vi "Regular Waves.vi"(0 "Run":bool, 1 "Wave Period":dbl(slide)=1.0 min=0.5 max=5.0 step=0.01 scale=0.5..5.0 scale format="%.1f", 2 "Wave Height":dbl(slide)=0.1 min=0.0 step=0.001 scale=0.0..0.15606733627984637 scale format="%.3f") -> ()   [LabVIEW 2012]
uses:
  <vilib>/DAQmx/write.llb/DAQmx Write (Analog 1D DBL 1Chan NSamp).vi
  <vilib>/DAQmx/write.llb/DAQmx Write (Analog 1D DBL NChan 1Samp).vi
  <vilib>/DAQmx/write.llb/DAQmx Write (Analog 2D DBL NChan NSamp).vi
  <vilib>/DAQmx/read.llb/DAQmx Read (Analog 2D DBL NChan NSamp).vi
  <vilib>/DAQmx/write.llb/DAQmx Write (Analog DBL 1Chan 1Samp).vi
  <vilib>/DAQmx/create/channels.llb/DAQmx Create Channel (AO-Voltage-Basic).vi
  <vilib>/DAQmx/configure/timing.llb/DAQmx Timing (Use Waveform).vi
  <vilib>/DAQmx/create/channels.llb/DAQmx Create Channel (AI-Voltage-Basic).vi
  <vilib>/DAQmx/configure/timing.llb/DAQmx Timing (Sample Clock).vi
  <vilib>/Analysis/1siggen.llb/Ramp Pattern by Samples.vi
  <vilib>/DAQmx/miscellaneous.llb/DAQmx Fill In Error Info.vi
  <vilib>/Analysis/NI_AALBase.lvlib
panel:
  out "Waveform Chart":dbl[][](graph)
  in  "Measure Waves":bool
  in  "Settings":bool
  in  "Power":bool
  out "Buffer Size":i32=4000
  # "Regular Wave Generator"
  # "s"
  # "m"
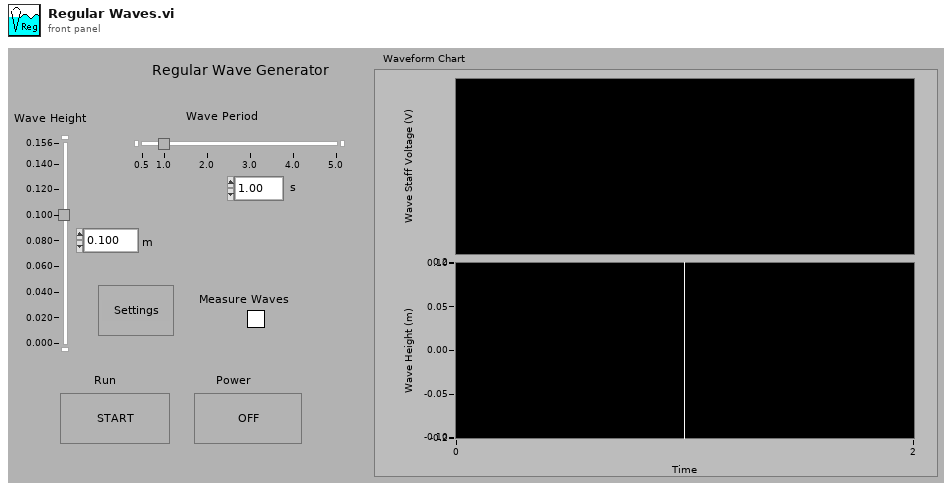
[diagram p1: front panel]
types:
  T1 = cluster{"Output Device":i16, "Output Channel":string, "Sampling Rate (Hz)":dbl, "Input Device":i16, "Input Channel":string, "Input Offset (V)":dbl, "Input Calibration (m/V)":dbl, "Stroke Calibration (V/m)":dbl, "Paddle Height (m)":dbl, "Water Depth (m)":dbl, "Min Period":dbl, "Max Period":dbl, "Max 1/2 Piston Stroke":dbl, "Max H/L":dbl, "Max H/d":dbl}
  T2 = cluster{"Period":dbl, "Wave Height":dbl, "Phase Angle (rad)":dbl}
  T3 = cluster{"Sampling Rate":i32, "Water Depth":dbl, "Paddle Height":dbl}
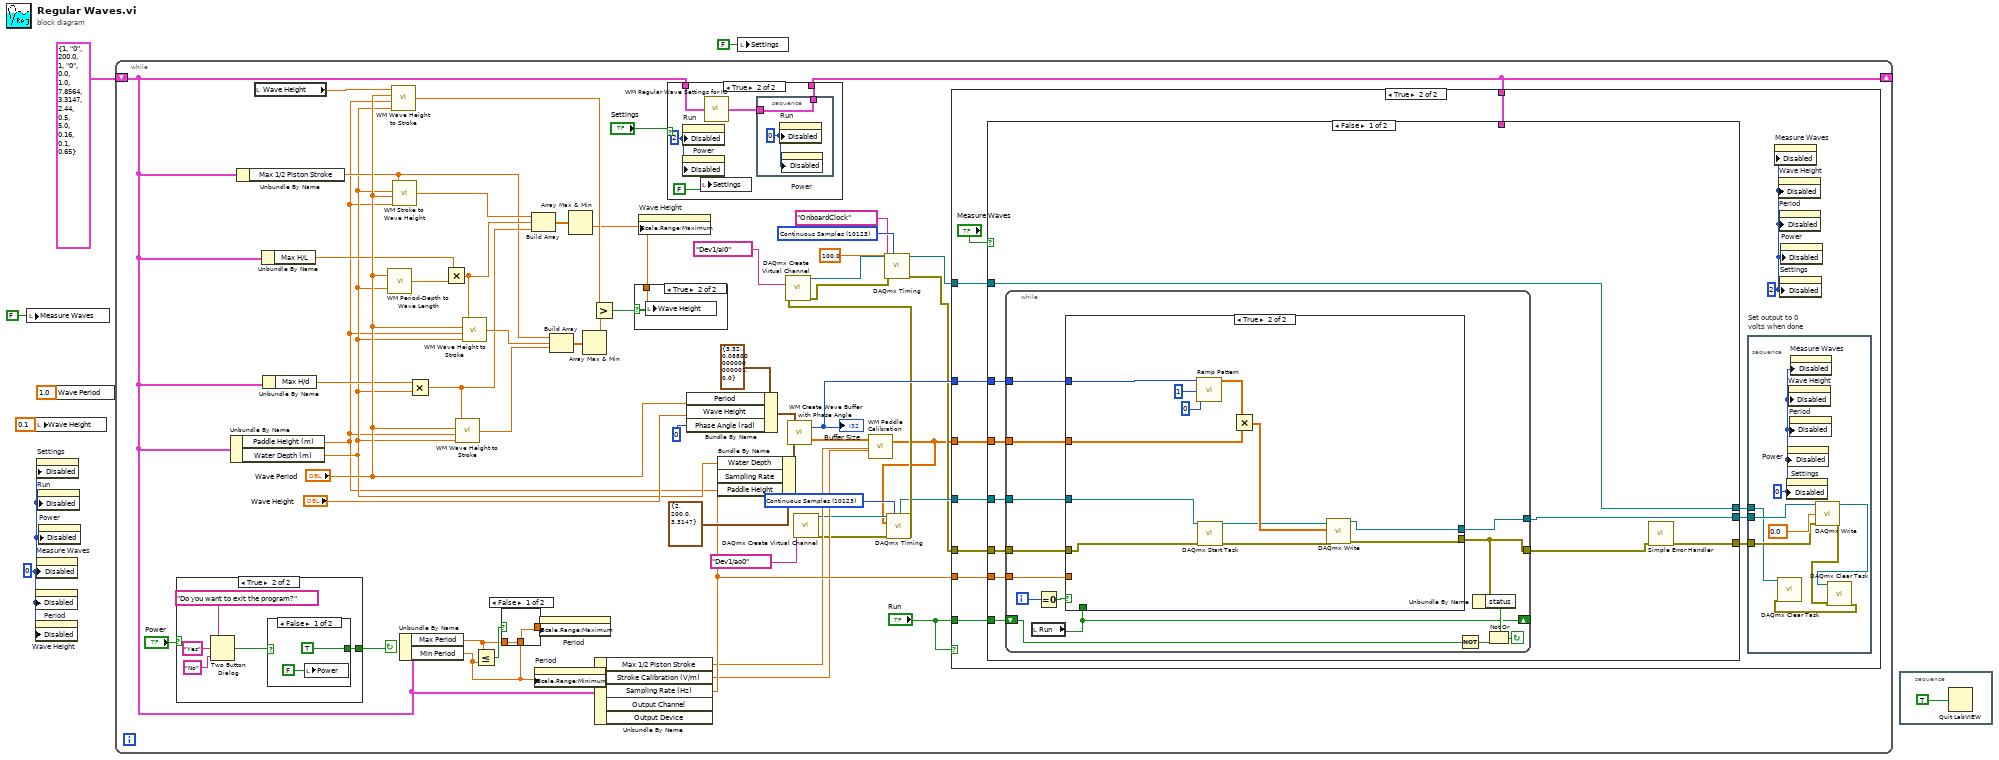
[diagram p0: block diagram]
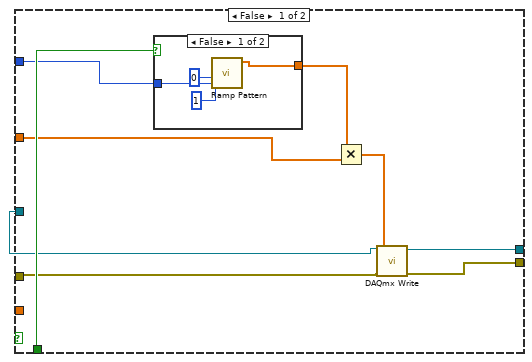
[diagram p3: hidden frame]
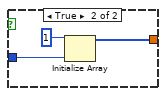
[diagram p4: hidden frame]
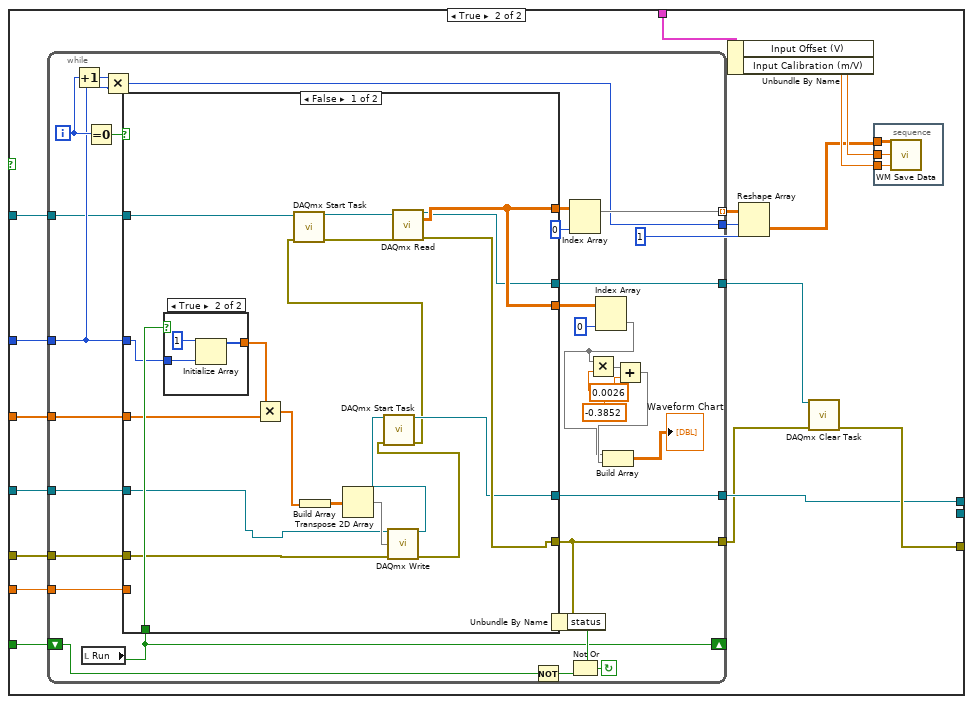
[diagram p5: hidden frame]
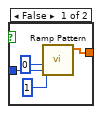
[diagram p6: hidden frame]
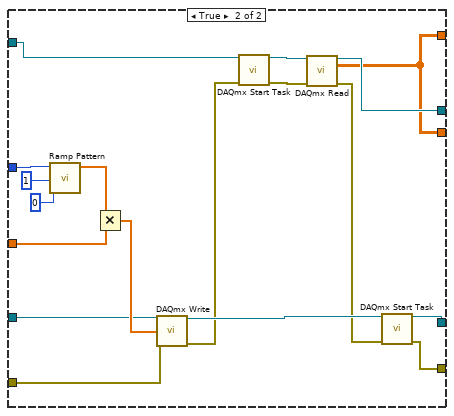
[diagram p7: hidden frame]
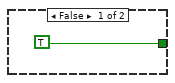
[diagram p9: hidden frame]
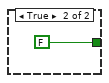
[diagram p10: hidden frame]
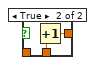
[diagram p11: hidden frame]
diagram:
  w2 = u8 0 ("Write Attribute")
  n1 = local write "Measure Waves"(FALSE ("Measure Waves")) -> ()
  n2 = local write "Wave Height"(0.1 ("Wave Height")) -> ()
  n3 = property on="Period" class="Slide (strict)"("Disabled"=w2) -> ()  [unwired: 2 in, 2 out]
  n4 = property on="Wave Height" class="Slide (strict)"("Disabled"=w2) -> ()  [unwired: 2 in, 2 out]
  n5 = property on="Measure Waves" class="Bool (strict)"("Disabled"=w2) -> ()  [unwired: 2 in, 2 out]
  n6 = property on="Settings" class="Bool (strict)"("Disabled"=w2) -> ()  [unwired: 2 in, 2 out]
  n7 = property on="Run" class="Bool (strict)"("Disabled"=w2) -> ()  [unwired: 2 in, 2 out]
  n8 = property on="Power" class="Bool (strict)"("Disabled"=w2) -> ()  [unwired: 2 in, 2 out]
  n9 = local write "Wave Period"(1.0 ("Period")) -> ()
  n10 = while {
    shift-left: T1 {"Output Device"=1, "Output Channel"="0", "Sampling Rate (Hz)"=200.0, "Input Device"=1, "Input Channel"="0", "Input Offset (V)"=0.0, "Input Calibration (m/V)"=1.0, "Stroke Calibration (V/m)"=7.8564, "Paddle Height (m)"=3.3147, "Water Depth (m)"=2.44, "Min Period"=0.5, "Max Period"=5.0, "Max 1/2 Piston Stroke"=0.16, "Max H/L"=0.1, "Max H/d"=0.65} ("Settings") -> [w27]
    shift-right: [w22] -> _
    stop <- w47 continue-if-true
    w9 = 10123 items=["Finite Samples"=10178, "Continuous Samples"=10123, "Hardware Timed Single Point"=12522] ("sample mode")
    w15 = 10123 items=["Finite Samples"=10178, "Continuous Samples"=10123, "Hardware Timed Single Point"=12522] ("sample mode")
    n11 = case shown="True" "Power" {
      tunnel: [TRUE w238] -> w47
      frame False {
      }
      frame True {
        n12 = Two Button Dialog(message="Do you want to exit the program?", 1:"No" ("F button name (\"Cancel\")"), 2:"Yes" ("T button name (\"OK\")")) -> (T button?=w239:bool)
        n13 = case shown="False" w239 {
          tunnel: [TRUE FALSE] -> w238
          frame False {
            n14 = local write "Power"(FALSE ("Power")) -> ()
          }
          frame True {
          }
        }
      }
    }
    n15 = Unbundle By Name(w27) -> ("Paddle Height (m)"=w30:dbl, "Water Depth (m)"=w31:dbl)
    n16 = Unbundle By Name(w27) -> ("Max 1/2 Piston Stroke"=w34:dbl)
    n17 = local read "Wave Height"() -> (w50:dbl)
    n18 = Unbundle By Name(w27) -> ("Max H/L"=w33:dbl)
    n19 = Unbundle By Name(w27) -> ("Max H/d"=w32:dbl)
    n20 = call "WM Period-Depth to Wave Length.vi"("Water Depth"=w31, "Period"="Wave Period") -> ("WaveLength"=w39:dbl)
    n21 = call "WM Wave Height to Stroke.vi"("Water Depth (m)"=w31, "Flap Height (m)"=w30, "Wave Period (s)"="Wave Period", "Wave Height (m)"=w50) -> ("Flap Amplitude (from x=0) (m)"=w59:dbl)
    n22 = call "WM Stroke to Wave Height.vi"("Paddle Height (m)"=w30, "Wave Period (s)"="Wave Period", "Water Depth (m)"=w31, "Flap Amplitude from x=0 (m)"=w34) -> ("Wave Height (m)"=w54:dbl)
    n23 = Unbundle By Name(w27) -> ("Max Period"=w26:dbl, "Min Period"=w25:dbl)
    n24 = Multiply(x=w32, y=w31) -> (x*y=w38:dbl)
    n25 = Multiply(x=w33, y=w39) -> (x*y=w55:dbl)
    n26 = call "WM Wave Height to Stroke.vi"("Water Depth (m)"=w31, "Flap Height (m)"=w30, "Wave Period (s)"="Wave Period", "Wave Height (m)"=w38) -> ("Flap Amplitude (from x=0) (m)"=w53:dbl)
    n27 = call "WM Wave Height to Stroke.vi"("Water Depth (m)"=w31, "Flap Height (m)"=w30, "Wave Period (s)"="Wave Period", "Wave Height (m)"=w55) -> ("Flap Amplitude (from x=0) (m)"=w52:dbl)
    n28 = Less Or Equal?(x=w26, y=w25) -> (x <= y?=w60:bool)
    n29 = case shown="False" w60 {
      tunnel: w25 -> [_ w248]
      tunnel: [w246 w247] -> w49
      tunnel: w26 -> [w246 _]
      frame False {
      }
      frame True {
        n30 = Increment(x=w248) -> (x+1=w247:dbl)
      }
    }
    n31 = Build Array(w54, w55, w38) -> (w58:dbl[])
    n32 = property on="Period" class="Slide (strict)"("Scale.Range:Minimum"=w25) -> ()  [unwired: 2 in, 2 out]
    n33 = property on="Period" class="Slide (strict)"("Scale.Range:Maximum"=w49) -> ()  [unwired: 2 in, 2 out]
    n34 = Build Array(w34, w52, w53) -> (w57:dbl[])
    n35 = Array Max & Min(array=w58) -> (min value=w51:dbl)  [unwired: 3 out]
    n36 = Array Max & Min(array=w57) -> (min value=w56:dbl)  [unwired: 3 out]
    n37 = Greater?(x=w59, y=w56) -> (0:w61:bool)
    n38 = Unbundle By Name(w27) -> ("Max 1/2 Piston Stroke"=w29:dbl, "Stroke Calibration (V/m)"=w28:dbl, "Sampling Rate (Hz)"=w35:dbl)  [unwired: 2 out]
    n39 = case shown="True" w61 {
      tunnel: w51 -> [_ w249]
      frame False {
      }
      frame True {
        n40 = local write "Wave Height"(w249) -> ()
      }
    }
    n41 = property on="Wave Height" class="Slide (strict)"("Scale.Range:Maximum"=w51) -> ()  [unwired: 2 in, 2 out]
    n42 = case shown="True" "Settings" {
      tunnel: w27 -> [w229 w234]
      tunnel: [w229 w232] -> w22
      frame False {
      }
      frame True {
        w230 = u8 2 ("Write Attribute")
        n43 = property on="Run" class="Bool (strict)"("Disabled"=w230) -> ()  [unwired: 2 in, 2 out]
        n44 = property on="Power" class="Bool (strict)"("Disabled"=w230) -> ()  [unwired: 2 in, 2 out]
        n45 = local write "Settings"(FALSE ("Settings")) -> ()
        n46 = call "WM Regular Wave Settings for IO.vi"("Settings"=w234) -> ("Settings Output"=w233:T1)
        n47 = stacked-sequence {
          tunnel: w233 -> [w236]
          tunnel: [w236] -> w232
          frame #0 {
            w235 = u8 0 ("Write Attribute")
            n48 = property on="Run" class="Bool (strict)"("Disabled"=w235) -> ()  [unwired: 2 in, 2 out]
            n49 = property on="Power" class="Bool (strict)"("Disabled"=w235) -> ()  [unwired: 2 in, 2 out]
          }
        }
      }
    }
    n50 = Bundle By Name(cluster=T2 {"Period"=3.32, "Wave Height"=0.08800000000000001, "Phase Angle (rad)"=0.0} ("Sine Paramaters"), "Period"="Wave Period", "Wave Height"="Wave Height", "Phase Angle (rad)"=0) -> (w42:T2)
    n51 = Bundle By Name(cluster=T3 {"Sampling Rate"=2, "Water Depth"=200.0, "Paddle Height"=3.3147} ("Buffer Info"), "Water Depth"=w31, "Sampling Rate"=w35, "Paddle Height"=w30) -> (w44:T3)
    n52 = call "WM Create Wave Buffer with Phase Angle.vi"("Buffer Info"=w44, "Sine Paramaters"=w42) -> ("Output"=w46:dbl[], "Buffer Size"=w24:i32)
    "Buffer Size" <- w24
    n53 = call-poly <vilib>:"DAQmx Create Virtual Channel.vi"("physical channels"=tag "Dev1/ao0") -> ("task out"=w19:refnum<k21>, "error out"=w18:errorcluster)  [unwired: 13 in]
    n54 = call "WM Paddle Calibration.vi"("Stroke Calibration (V/m)"=w28, "Max 1/2 Piston Stroke (m)"=w29, "Input Stroke Distance (m)"=w46) -> ("Output Voltage"=w7:dbl[])  [unwired: 1 in, 1 out]
    n55 = call-poly <vilib>:"DAQmx Timing.vi"("task/channels in"=w19, "sample mode"=w15, "waveform"=w7, "error in"=w18) -> ("task out"=w16:refnum<k21>, "error out"=w17:errorcluster)  [unwired: 10 in]
    n56 = call-poly <vilib>:"DAQmx Create Virtual Channel.vi"("physical channels"=tag "Dev1/ai0", "error in"=w17) -> ("task out"=w14:refnum<k21>, "error out"=w11:errorcluster)  [unwired: 12 in]
    n57 = call-poly <vilib>:"DAQmx Timing.vi"("task/channels in"=w14, "sample mode"=w9, "rate"=100.0, "source"=tag "OnboardClock", "error in"=w11) -> ("task out"=w13:refnum<k21>, "error out"=w12:errorcluster)  [unwired: 9 in]
    n58 = case shown="True" "Run" {
      tunnel: w24 -> [_ w73]
      tunnel: "Run" -> [_ w72]
      tunnel: w7 -> [_ w71]
      tunnel: w35 -> [_ w70]
      tunnel: w22 -> [_ w67]
      tunnel: w16 -> [_ w66]
      tunnel: w12 -> [_ w65]
      tunnel: w13 -> [_ w64]
      frame False {
      }
      frame True {
        w68 = u8 2 ("Write Attribute")
        n59 = case shown="False" "Measure Waves" {
          tunnel: [w84 w129] -> w74
          tunnel: w73 -> [w83 w144]
          tunnel: w72 -> [w82 w142]
          tunnel: w71 -> [w81 w143]
          tunnel: w70 -> [w80 w141]
          tunnel: w67 -> [_ w140]
          tunnel: w66 -> [w79 w133]
          tunnel: w65 -> [w78 w132]
          tunnel: w64 -> [w77 w131]
          tunnel: [w77 w128] -> w63
          tunnel: [w75 _] -> w62
          frame False {
            n60 = while {
              tunnel: [w89] -> w76
              tunnel: w83 -> [w90]
              tunnel: w81 -> [w91]
              tunnel: w80 -> [w92]
              shift-left: w82 -> [w93]
              shift-right: [w88] -> _
              tunnel: w79 -> [w87]
              tunnel: w78 -> [w86]
              tunnel: [w85] -> w75
              i -> [w98]
              stop <- w94 continue-if-true
              n61 = local read "Run"() -> (w88:bool)
              n62 = Equal To 0?(x=w98) -> (x = 0?=w97:bool)
              n63 = case shown="True" w97 {
                tunnel: [w99 w115] -> w89
                tunnel: w92 -> [_ _]
                tunnel: w88 -> [w106 _]
                tunnel: w91 -> [w105 w122]
                tunnel: w90 -> [w104 w123]
                tunnel: w87 -> [w101 w120]
                tunnel: w86 -> [w100 w119]
                tunnel: [w103 w116] -> w85
                frame False {
                  n64 = case shown="False" w106 {
                    tunnel: [w111 w112] -> w107
                    tunnel: w104 -> [w108 w114]
                    frame False {
                      n65 = call-poly <vilib>:"Ramp Pattern.vi"("start"=1, "end"=0, "samples"=w108) -> ("Ramp Pattern"=w111:dbl[])  [unwired: 7 in, 1 out]
                    }
                    frame True {
                      n66 = Initialize Array(1, w114) -> (w112:i32[])
                    }
                  }
                  n67 = Multiply(x=w107, y=w105) -> (x*y=w102:dbl[])
                  n68 = call-poly <vilib>:"DAQmx Write.vi"("task/channels in"=w101, "data"=w102, "error in"=w100) -> ("task out"=w103:refnum<k21>, "error out"=w99:errorcluster)  [unwired: 10 in, 1 out]
                }
                frame True {
                  n69 = call-poly <vilib>:"Ramp Pattern.vi"("start"=0, "end"=1, "samples"=w123) -> ("Ramp Pattern"=w124:dbl[])  [unwired: 7 in, 1 out]
                  n70 = call <vilib>:"DAQmx Start Task.vi"("task/channels in"=w120, "error in"=w119) -> ("task out"=w118:refnum<k21>, "error out"=w117:errorcluster)  [unwired: 12 in]
                  n71 = Multiply(x=w124, y=w122) -> (x*y=w121:dbl[])
                  n72 = call-poly <vilib>:"DAQmx Write.vi"("task/channels in"=w118, "data"=w121, "error in"=w117) -> ("task out"=w116:refnum<k21>, "error out"=w115:errorcluster)  [unwired: 10 in, 1 out]
                }
              }
              n73 = Not(x=w93) -> (.not. x?=w95:bool)
              n74 = Unbundle By Name(w89) -> ("status"=w96:bool)
              n75 = Not Or(1:w95, 2:w96) -> (0:w94:bool)
            }
            n76 = call <vilib>:"Simple Error Handler.vi"("error in (no error)"=w76) -> ("error out"=w84:errorcluster)  [unwired: 4 in, 4 out]
          }
          frame True {
            n77 = while {
              tunnel: [w158] -> w135
              tunnel: [w163] -> w137 mode=indexing
              tunnel: [w165] -> w127
              tunnel: w144 -> [w159]
              tunnel: w143 -> [w167]
              tunnel: w141 -> [w168]
              shift-left: w142 -> [w169]
              shift-right: [w166] -> _
              tunnel: w133 -> [w149]
              tunnel: w132 -> [w148]
              tunnel: w131 -> [w147]
              tunnel: [w146] -> w128
              tunnel: [w145] -> w130
              i -> [w161]
              stop <- w170 continue-if-true
              n78 = Increment(x=w161) -> (x+1=w160:i32)
              n79 = local read "Run"() -> (w166:bool)
              n80 = Equal To 0?(x=w161) -> (x = 0?=w173:bool)
              n81 = Multiply(x=w160, y=w159) -> (x*y=w158:i32)
              n82 = case shown="False" w173 {
                tunnel: [w184 w200] -> w165
                tunnel: w168 -> [_ _]
                tunnel: w166 -> [w191 _]
                tunnel: w167 -> [w189 w214]
                tunnel: w159 -> [w187 w213]
                tunnel: [w185 w205] -> w164
                tunnel: [w185 w205] -> w153
                tunnel: w149 -> [w177 w211]
                tunnel: w148 -> [w176 w210]
                tunnel: w147 -> [w174 w201]
                tunnel: [w180 w208] -> w146
                tunnel: [w183 w206] -> w145
                frame False {
                  n83 = case shown="True" w191 {
                    tunnel: [w196 w197] -> w192
                    tunnel: w187 -> [w193 w199]
                    frame False {
                      n84 = call-poly <vilib>:"Ramp Pattern.vi"("start"=1, "end"=0, "samples"=w193) -> ("Ramp Pattern"=w196:dbl[])  [unwired: 7 in, 1 out]
                    }
                    frame True {
                      n85 = Initialize Array(1, w199) -> (w197:i32[])
                    }
                  }
                  n86 = Multiply(x=w192, y=w189) -> (x*y=w188:dbl[])
                  n87 = Build Array(w188) -> (w190:dbl[][])
                  n88 = Transpose 2D Array(2D array=w190) -> (transposed array=w186:dbl[][])
                  n89 = call-poly <vilib>:"DAQmx Write.vi"("task/channels in"=w177, "data"=w186, "error in"=w176) -> ("task out"=w181:refnum<k21>, "error out"=w182:errorcluster)  [unwired: 10 in, 1 out]
                  n90 = call <vilib>:"DAQmx Start Task.vi"("task/channels in"=w181, "error in"=w182) -> ("task out"=w180:refnum<k21>, "error out"=w175:errorcluster)  [unwired: 12 in]
                  n91 = call <vilib>:"DAQmx Start Task.vi"("task/channels in"=w174, "error in"=w175) -> ("task out"=w179:refnum<k21>, "error out"=w178:errorcluster)  [unwired: 12 in]
                  n92 = call-poly <vilib>:"DAQmx Read.vi"("task/channels in"=w179, "error in"=w178) -> ("task out"=w183:refnum<k21>, "data"=w185:dbl[][], "error out"=w184:errorcluster)  [unwired: 11 in]
                }
                frame True {
                  n93 = call-poly <vilib>:"Ramp Pattern.vi"("start"=0, "end"=1, "samples"=w213) -> ("Ramp Pattern"=w215:dbl[])  [unwired: 7 in, 1 out]
                  n94 = Multiply(x=w215, y=w214) -> (x*y=w212:dbl[])
                  n95 = call-poly <vilib>:"DAQmx Write.vi"("task/channels in"=w211, "data"=w212, "error in"=w210) -> ("task out"=w209:refnum<k21>, "error out"=w207:errorcluster)  [unwired: 10 in, 1 out]
                  n96 = call <vilib>:"DAQmx Start Task.vi"("task/channels in"=w201, "error in"=w207) -> ("task out"=w204:refnum<k21>, "error out"=w203:errorcluster)  [unwired: 12 in]
                  n97 = call-poly <vilib>:"DAQmx Read.vi"("task/channels in"=w204, "error in"=w203) -> ("task out"=w206:refnum<k21>, "data"=w205:dbl[][], "error out"=w202:errorcluster)  [unwired: 11 in]
                  n98 = call <vilib>:"DAQmx Start Task.vi"("task/channels in"=w209, "error in"=w202) -> ("task out"=w208:refnum<k21>, "error out"=w200:errorcluster)  [unwired: 12 in]
                }
              }
              n99 = Not(x=w169) -> (.not. x?=w171:bool)
              n100 = Unbundle By Name(w165) -> ("status"=w172:bool)
              n101 = Index Array(array=w164, index (col)=0 ("Index")) -> (element=w163:dbl[])  [unwired: 1 in]
              n102 = Not Or(1:w171, 2:w172) -> (0:w170:bool)
              n103 = Index Array(array=w153, index (col)=0 ("disabled index (col)")) -> (element=w151:dbl[])  [unwired: 1 in]
              n104 = Multiply(x=w151, y=-0.3852) -> (x*y=w156:dbl[])
              n105 = Add(x=w156, y=0.0026) -> (x+y=w152:dbl[])
              n106 = Build Array(w151, w152) -> (→"Waveform Chart":dbl[][])
            }
            n107 = Unbundle By Name(w140) -> ("Input Offset (V)"=w139:dbl, "Input Calibration (m/V)"=w138:dbl)
            n108 = Reshape Array(w137, w135, 1 ("Dimension Size")) -> (w136:dbl[][])
            n109 = call <vilib>:"DAQmx Clear Task.vi"("task in"=w130, "error in"=w127) -> ("error out"=w129:errorcluster)  [unwired: 13 in]
            n110 = stacked-sequence {
              tunnel: w136 -> [w220]
              tunnel: w139 -> [w219]
              tunnel: w138 -> [w218]
              frame #0 {
                n111 = call "WM Save Data.vi"("Input Calibration"=w218, "Input Offset"=w219, "Input Data"=w220) -> ()
              }
            }
          }
        }
        n112 = stacked-sequence "Set output to 0\nvolts when done" {
          tunnel: w74 -> [w226]
          tunnel: w63 -> [w222]
          tunnel: w62 -> [w223]
          frame #0 {
            w228 = u8 0 ("Write Attribute")
            n113 = property on="Settings" class="Bool (strict)"("Disabled"=w228) -> ()  [unwired: 2 in, 2 out]
            n114 = property on="Power" class="Bool (strict)"("Disabled"=w228) -> ()  [unwired: 2 in, 2 out]
            n115 = property on="Wave Height" class="Slide (strict)"("Disabled"=w228) -> ()  [unwired: 2 in, 2 out]
            n116 = property on="Period" class="Slide (strict)"("Disabled"=w228) -> ()  [unwired: 2 in, 2 out]
            n117 = property on="Measure Waves" class="Bool (strict)"("Disabled"=w228) -> ()  [unwired: 2 in, 2 out]
            n118 = call-poly <vilib>:"DAQmx Write.vi"("task/channels in"=w223, "data"=sgl 0.0 ("Set analog output to 0"), "error in"=w226) -> ("task out"=w224:refnum<k21>, "error out"=w225:errorcluster)  [unwired: 10 in, 1 out]
            n119 = call <vilib>:"DAQmx Clear Task.vi"("task in"=w224, "error in"=w225) -> ("error out"=w221:errorcluster)  [unwired: 13 in]
            n120 = call <vilib>:"DAQmx Clear Task.vi"("task in"=w222, "error in"=w221) -> ()  [unwired: 13 in, 1 out]
          }
        }
        n121 = property on="Measure Waves" class="Bool (strict)"("Disabled"=w68) -> ()  [unwired: 2 in, 2 out]
        n122 = property on="Wave Height" class="Slide (strict)"("Disabled"=w68) -> ()  [unwired: 2 in, 2 out]
        n123 = property on="Period" class="Slide (strict)"("Disabled"=w68) -> ()  [unwired: 2 in, 2 out]
        n124 = property on="Settings" class="Bool (strict)"("Disabled"=w68) -> ()  [unwired: 2 in, 2 out]
        n125 = property on="Power" class="Bool (strict)"("Disabled"=w68) -> ()  [unwired: 2 in, 2 out]
      }
    }
  }
  n126 = local write "Settings"(FALSE ("Settings")) -> ()
  n127 = stacked-sequence {
    frame #0 {
      n128 = Quit LabVIEW(quit? (T)=TRUE) -> ()
    }
  }
